vi "Initialise State.vi"(8 "error in (no error)":errorcluster, 11 "OnChange_Boolean in":refnum<class "OnChangeNotifier_Boolean.lvclass">) -> (0 "error out":errorcluster, 3 "OnChange_Boolean out":refnum<class "OnChangeNotifier_Boolean.lvclass">)   [LabVIEW 2021, in "OnChangeNotifier_Boolean.lvclass"]
uses:
  OnChangeNotifier_Boolean.lvclass
  OnChangeNotifier_Boolean.lvclass/OnChangeNotifier_Boolean.ctl
  <vilib>/TSA/Abstract Data Classes/Abs_Types/Boolean/Abs_Boolean.lvclass
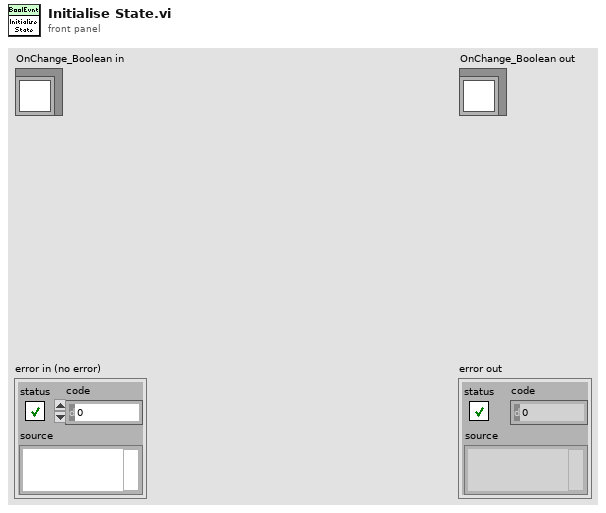
[diagram p1: front panel]
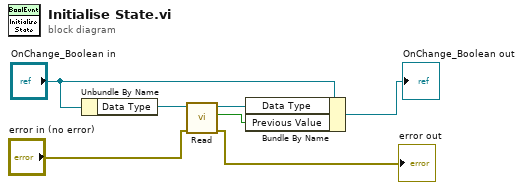
[diagram p0: block diagram]
diagram:
  n1 = Unbundle By Name("OnChange_Boolean in") -> ("Data Type"=w7:refnum<class "Abs_Boolean.lvclass">)
  n2 = call-dynamic "Read.vi"("error in (no error)"="error in (no error)", "Boolean in"=w7) -> ("error out"=→"error out":errorcluster, "Boolean"=w3:bool, "Boolean out"=w5:refnum<class "Abs_Boolean.lvclass">)  [unwired: 7 in]
  n3 = Bundle By Name(cluster="OnChange_Boolean in", "Data Type"=w5, "Previous Value"=w3) -> (→"OnChange_Boolean out":refnum<class "OnChangeNotifier_Boolean.lvclass">)
